vi "params.vi"() -> ()   [LabVIEW 2015]
uses:
  type def/NI card channels.ctl
  type def/NI tasks.ctl
panel:
  in  "task status":refnum<vi>
  in  "task plan":refnum<vi>
  out "NI tasks":T1
  in  "y flyback pixel":u16
  in  "PXI channel":refnum<vi>
  in  "x flyback pixel":u16
  in  "advanced params":refnum<vi>
  in  "basic params":refnum<vi>
  in  "current state":refnum<vi>
  in  "imaging mode":refnum<vi>
  in  "NI card channels":T2
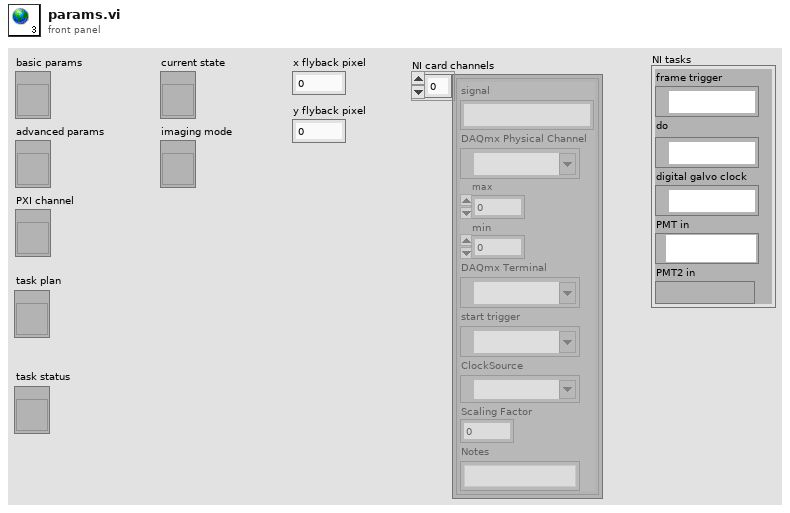
[diagram p1: front panel]
types:
  T1 = typedef "NI tasks.ctl" = cluster{"frame trigger":refnum<k21>, "do":refnum<k21>, "digital galvo clock":refnum<k21>, "PMT in":refnum<k15>, "PMT2 in":refnum<k15>}
  T2 = typedef "NI card channels.ctl" = cluster{"signal":string, "DAQmx Physical Channel":tag, "max":dbl, "min":dbl, "DAQmx Terminal":tag, "start trigger":tag, "ClockSource":tag, "Scaling Factor":dbl, "Notes":string}[]
diagram:
